vi "test3-SafeStr conversion.vi"(8 "error in (no error)":errorcluster, 11 "TestCase in":refnum<class "testcase-CSMArgument.lvclass">) -> (0 "error out":errorcluster, 3 "TestCase out":refnum<class "testcase-CSMArgument.lvclass">)   [LabVIEW 2017, in "testcase-CSMArgument.lvclass"]
uses:
  testcase-CSMArgument.lvclass
  src/user.lib/_NEVSTOP/Communicable State Machine(CSM)/AdvanceAPI/CSM - Keywords.vi
  src/user.lib/_NEVSTOP/Communicable State Machine(CSM)/_Shared/Trim Single-line Text.vi
  <vilib>/addons/_JKI Toolkits/VI Tester/TestCase.llb/TestCase.lvclass
  src/user.lib/_NEVSTOP/Communicable State Machine(CSM)/Communicable State Machine.lvlib
  src/user.lib/_NEVSTOP/Communicable State Machine(CSM)/_Shared/CSM Shared.lvlib
  C:/Program Files (x86)/National Instruments/LabVIEW 2017/vi.lib/addons/_JKI Toolkits/VI Tester/TestCase.llb/TestCase.lvclass
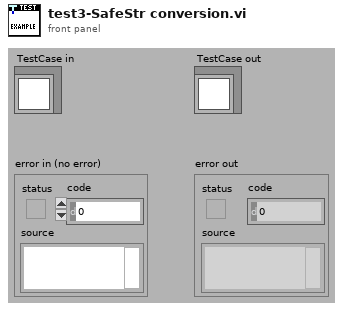
[diagram p1: front panel]
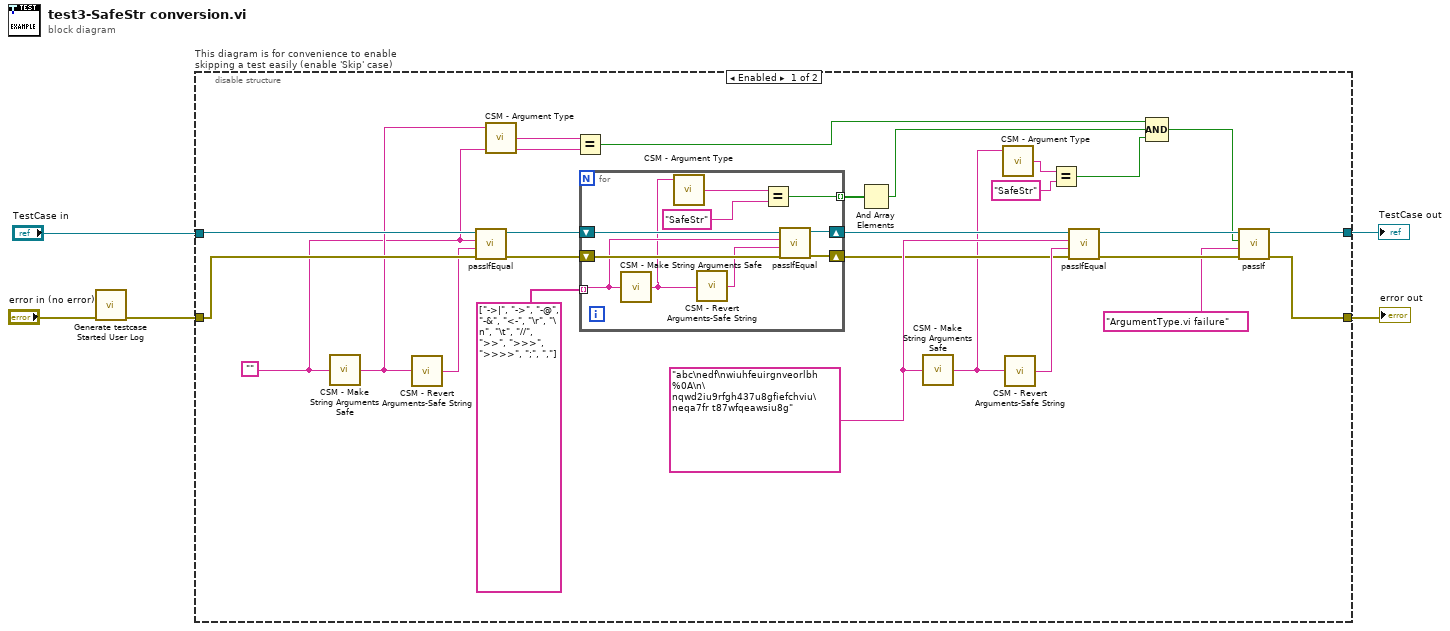
[diagram p0: block diagram]
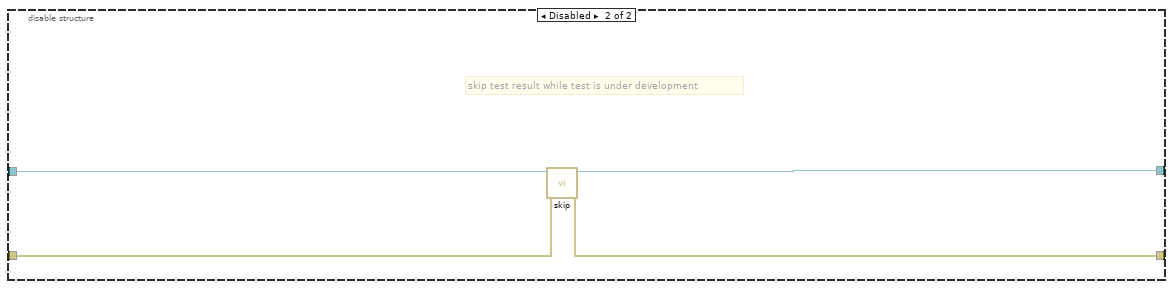
[diagram p2: hidden frame]
diagram:
  n1 = call "Generate testcase Started User Log.vi"("Error In"="error in (no error)") -> ("error out"=w1:errorcluster)  [unwired: 10 in]
  n2 = disable-structure "This diagram is for convenience to enable skipping a test easily (enable 'Skip' case)" shown="Enabled" {
    disable-tunnel: "TestCase in" -> [w31 w45]
    disable-tunnel: [w14 w43] -> w2
    disable-tunnel: [w16 w44] -> w4
    disable-tunnel: w1 -> [w30 w42]
    frame Enabled {
      w24 = "abc\nedf\nwiuhfeuirgnveorlbh %0A\n\nqwd2iu9rfgh437u8gfiefchviu\neqa7fr t87wfqeawsiu8g"
      w6 = ""
      n3 = call "CSM - Make String Arguments Safe.vi"("Argument String"=w6) -> ("Safe Argument String"=w7:string)  [unwired: 8 in]
      n4 = call "CSM - Revert Arguments-Safe String.vi"("Safe Argument String"=w7) -> ("Origin Argument String"=w29:string)  [unwired: 8 in]
      n5 = call-dynamic "passIfEqual.vi"("error in (no error)"=w30, "y"=w29, "x"=w6, "TestCase in"=w31) -> ("error out"=w26:errorcluster, "TestCase out"=w27:refnum<class "testcase-CSMArgument.lvclass">)  [unwired: 6 in]
      n6 = call "CSM - Argument Type.vi"("Arguments"=w7) -> ("Argument Type"=w21:string)  [unwired: 3 in, 1 out]
      n7 = Equal?(x=w21, y=w6) -> (x = y?=w13:bool)
      n8 = for {
        tunnel: string[] ["->|", "->", "-@", "-&", "<-", "\r", "\n", "\t", "//", ">>", ">>>", ">>>>", ";", ","] -> [w37] mode=indexing
        shift-right: [w40] -> w23
        shift-left: w27 -> [w41]
        shift-right: [w38] -> w22
        shift-left: w26 -> [w39]
        tunnel: [w32] -> w11 mode=indexing
        n9 = call "CSM - Make String Arguments Safe.vi"("Argument String"=w37) -> ("Safe Argument String"=w34:string)  [unwired: 8 in]
        n10 = call "CSM - Argument Type.vi"("Arguments"=w34) -> ("Argument Type"=w35:string)  [unwired: 3 in, 1 out]
        n11 = call "CSM - Revert Arguments-Safe String.vi"("Safe Argument String"=w34) -> ("Origin Argument String"=w36:string)  [unwired: 8 in]
        n12 = Equal?(x=w35, y="SafeStr") -> (x = y?=w32:bool)
        n13 = call-dynamic "passIfEqual.vi"("error in (no error)"=w39, "y"=w36, "x"=w37, "TestCase in"=w41) -> ("error out"=w38:errorcluster, "TestCase out"=w40:refnum<class "testcase-CSMArgument.lvclass">)  [unwired: 6 in]
      }
      n14 = And Array Elements(Boolean array=w11) -> (logical AND=w10:bool)
      n15 = call "CSM - Make String Arguments Safe.vi"("Argument String"=w24) -> ("Safe Argument String"=w20:string)  [unwired: 8 in]
      n16 = call "CSM - Argument Type.vi"("Arguments"=w20) -> ("Argument Type"=w19:string)  [unwired: 3 in, 1 out]
      n17 = call "CSM - Revert Arguments-Safe String.vi"("Safe Argument String"=w20) -> ("Origin Argument String"=w25:string)  [unwired: 8 in]
      n18 = Equal?(x=w19, y="SafeStr") -> (x = y?=w12:bool)
      n19 = call-dynamic "passIfEqual.vi"("error in (no error)"=w22, "y"=w25, "x"=w24, "TestCase in"=w23) -> ("error out"=w17:errorcluster, "TestCase out"=w15:refnum<class "testcase-CSMArgument.lvclass">)  [unwired: 6 in]
      n20 = Compound Arithmetic op=AND(w13, w10, w12) -> (w9:bool)
      n21 = call-dynamic "passIf.vi"("error in (no error)"=w17, "message (\"\")"="ArgumentType.vi failure" ("message (\"\")"), "pass"=w9, "TestCase in"=w15) -> ("error out"=w16:errorcluster, "TestCase out"=w14:refnum<class "testcase-CSMArgument.lvclass">)  [unwired: 6 in]
    }
    frame Disabled {
      # "skip test result while test is under development"
      n22 = call <vilib>:"skip.vi"("error in (no error)"=w42, "TestCase in"=w45) -> ("error out"=w44:errorcluster, "TestCase out"=w43:refnum<class "testcase-CSMArgument.lvclass">)  [unwired: 8 in]
    }
  }
  "error out" <- w4
  "TestCase out" <- w2
